vi "XYZ Stage-Command request module.vi"(8 "error in":errorcluster, 9 "Command":T2=enum."Initialize", 11 "XYZ Stage data to queue":T1={"Command"=enum."Initialize", "Channel"="Z", "X"=0.0, "Y"=0.0, "Z"=0.0, "Speed"=0, "Zero"=FALSE, "Use acknowledgement?"=TRUE} {"Speed" format="Speed= %.0f"; "Z" format="Z= %#_g"; "Y" format="Y= %#_g"; "X" format="X= %#_g"}) -> (0 "error out":errorcluster, 1 "Timed out while waiting for acknowledgement":bool, 2 "Dequeue timed out":bool, 3 "XYZ Stage dequeued data":T1={"Command"=enum."Initialize", "Channel"="Z", "X"=0.0, "Y"=0.0, "Z"=0.0, "Speed"=0, "Zero"=FALSE, "Use acknowledgement?"=TRUE} {"Speed" format="Speed= %.0f"; "Z" format="Z= %#_g"; "Y" format="Y= %#_g"; "X" format="X= %#_g"}, 4 "Acknowledgement message":string)   [LabVIEW 2013]
doc: "This is the interface module handling all inter-process signaling between the main software and the XYZ stage driver."
uses:
  Typedefs/XYZ stage data.ctl
  Typedefs/XYZ stage states.ctl
  Typedefs/XYZ channel ring.ctl
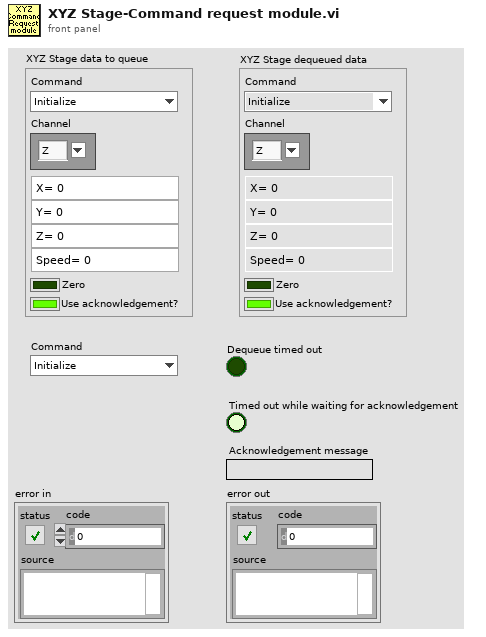
[diagram p1: front panel]
types:
  T1 = typedef "XYZ stage data.ctl" = cluster{"Command":T2, "Channel":T3, "X":sgl, "Y":sgl, "Z":sgl, "Speed":i32, "Zero":bool, "Use acknowledgement?":bool}
  T2 = typedef "XYZ stage states.ctl" = enum16{"Dequeue", "Initialize", "Read Position", "Read Speed Setting", "Move", "Set Max Speed", "Reset Axis", "Stop all movement"}
  T3 = typedef "XYZ channel ring.ctl" = string
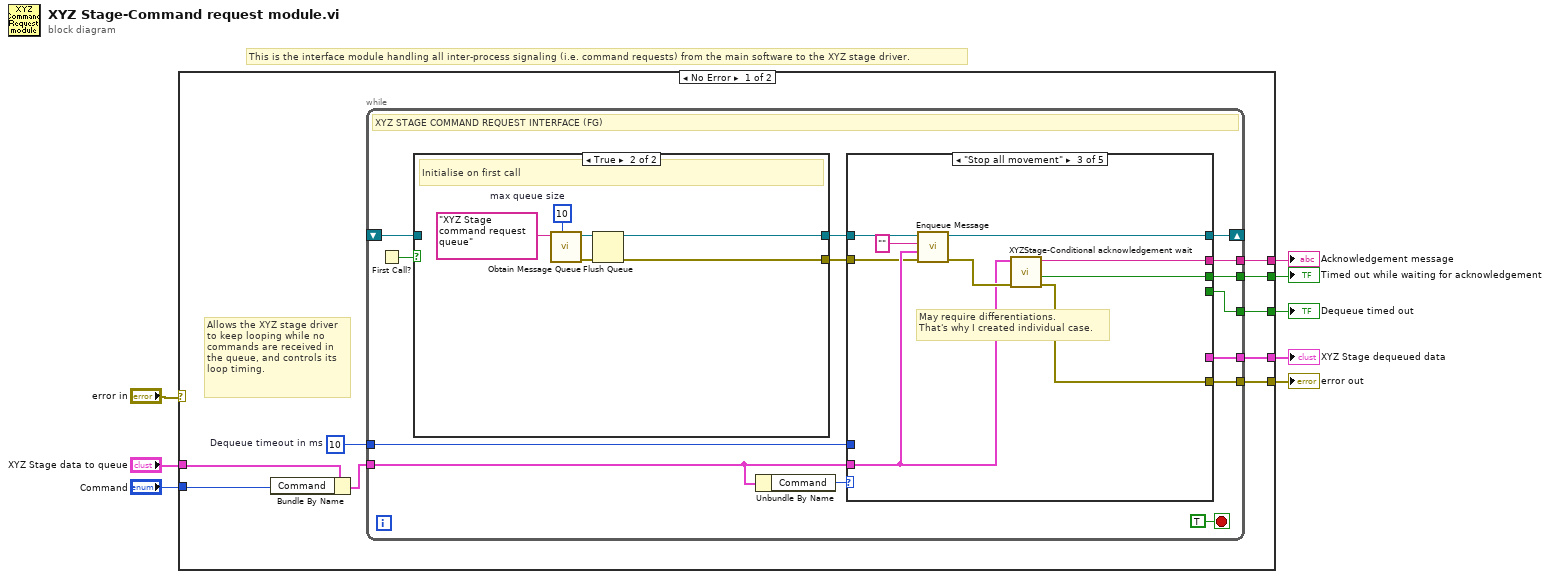
[diagram p0: block diagram]
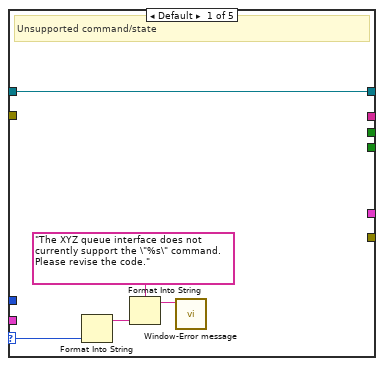
[diagram p2: hidden frame]
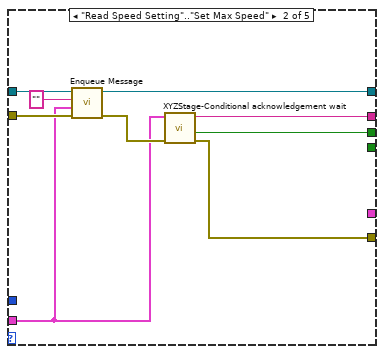
[diagram p3: hidden frame]
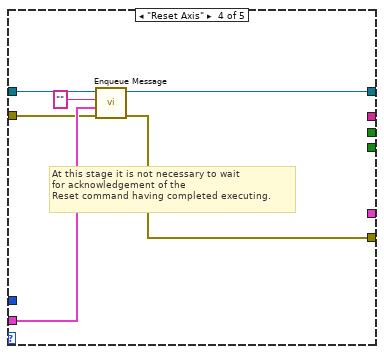
[diagram p4: hidden frame]
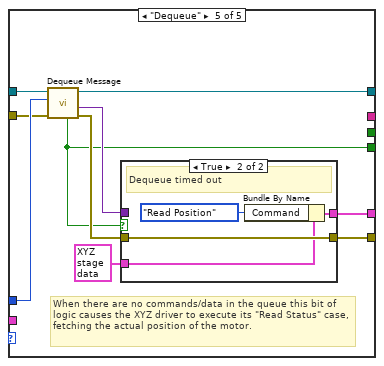
[diagram p5: hidden frame]
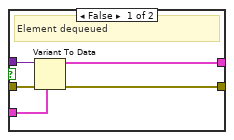
[diagram p6: hidden frame]
diagram:
  # "This is the interface module handling all inter-process signaling (i.e. command requests) from the main software to the XYZ stage driver."
  n1 = case shown="No Error" "error in" {
    selector: "error in" -> [_ w87]
    tunnel: "XYZ Stage data to queue" -> [w16 _]
    tunnel: "Command" -> [w15 _]
    tunnel: [w14 _] -> w6
    tunnel: [w13 _] -> w5
    tunnel: [w12 w87] -> w4
    tunnel: [w11 _] -> w2
    tunnel: [w10 _] -> w1
    frame No Error {
      w9 = 10  # Dequeue timeout in ms
      # "Allows the XYZ stage driver to keep looping while no commands are received in the queue, and controls its loop timing."
      n2 = Bundle By Name(cluster=w16, "Command"=w15) -> (w17:T1)
      n3 = while {
        shift-right: [w25] -> _
        shift-left: _ -> [w29]
        tunnel: w17 -> [w26]
        tunnel: [w24] -> w14
        tunnel: [w23] -> w13
        tunnel: w9 -> [w22]
        tunnel: [w20] -> w12
        tunnel: [w19] -> w11
        tunnel: [w18] -> w10
        stop <- TRUE stop-if-true
        # "XYZ STAGE COMMAND REQUEST INTERFACE (FG)"
        n4 = First Call?() -> (First Call?: T/F=w30:bool)
        n5 = case shown="True" w30 {
          tunnel: [w80 w83] -> w28
          tunnel: w29 -> [w80 _]
          tunnel: [_ w82] -> w21
          frame False {
          }
          frame True {
            w84 = 10  # max queue size
            # "Initialise on first call"
            n6 = call "Obtain Message Queue.vi"("max queue size (-1, unlimited)"=w84, "Queue name"="XYZ Stage command request queue") -> ("error out"=w85:errorcluster, "Message Queue"=w86:refnum<queue>)  [unwired: 8 in]
            n7 = Flush Queue(queue=w86, error in (no error)=w85) -> (queue out=w83:refnum<queue>, error out=w82:errorcluster)  [unwired: 1 out]
          }
        }
        n8 = Unbundle By Name(w26) -> ("Command"=w27:T2)
        n9 = case shown="\"Stop all movement\"" w27 {
          selector: w27 -> [w35 _ _ _ _]
          tunnel: w28 -> [w36 w45 w47 w60 w70]
          tunnel: w26 -> [_ w38 w49 w59 _]
          tunnel: [w36 w44 w54 w58 w68] -> w25
          tunnel: [_ _ _ _ w61] -> w24
          tunnel: [_ _ _ _ w62] -> w23
          tunnel: w22 -> [_ _ _ _ w67]
          tunnel: w21 -> [_ w42 w46 w56 w66]
          tunnel: [_ w40 w51 w55 w64] -> w20
          tunnel: [_ w37 w48 _ _] -> w19
          tunnel: [_ w39 w50 _ _] -> w18
          frame Default {
            # "Unsupported command/state"
            n10 = Format Into String(w35) -> (resulting string=w33:string)  [unwired: 3 in, 1 out]
            n11 = Format Into String(format string="The XYZ queue interface does not currently support the \"%s\" command. Please revise the code.", w33) -> (resulting string=w32:string)  [unwired: 2 in, 1 out]
            n12 = call "Window-Error message.vi"("Message"=w32) -> ()  [unwired: 10 in, 1 out]
          }
          frame "Read Speed Setting".."Set Max Speed" {
            n13 = call "Enqueue Message.vi"("error in (no error)"=w42, "Message Data"=w38, "Message"="", "Queue"=w45) -> ("error out"=w41:errorcluster, "Queue out"=w44:refnum<queue>)  [unwired: 6 in]
            n14 = call "XYZStage-Conditional acknowledgement wait.vi"("error in (no error)"=w41, "XYZ Stage data to queue"=w38) -> ("error out"=w40:errorcluster, "Timed out while waiting for acknowledgement"=w37:bool, "Acknowledgement Message out"=w39:string)  [unwired: 7 in]
          }
          frame "Stop all movement" {
            # "May require differentiations.\nThat's why I created individual case."
            n15 = call "Enqueue Message.vi"("error in (no error)"=w46, "Message Data"=w49, "Message"="", "Queue"=w47) -> ("error out"=w52:errorcluster, "Queue out"=w54:refnum<queue>)  [unwired: 6 in]
            n16 = call "XYZStage-Conditional acknowledgement wait.vi"("error in (no error)"=w52, "XYZ Stage data to queue"=w49) -> ("error out"=w51:errorcluster, "Timed out while waiting for acknowledgement"=w48:bool, "Acknowledgement Message out"=w50:string)  [unwired: 7 in]
          }
          frame "Reset Axis" {
            # "At this stage it is not necessary to wait \nfor acknowledgement of the\nReset command having completed executing."
            n17 = call "Enqueue Message.vi"("error in (no error)"=w56, "Message Data"=w59, "Message"="", "Queue"=w60) -> ("error out"=w55:errorcluster, "Queue out"=w58:refnum<queue>)  [unwired: 6 in]
          }
          frame "Dequeue" {
            # "When there are no commands/data in the queue this bit of logic causes the XYZ driver to execute its \"Read Status\" case, fetching the actual position of the motor."
            n18 = call "Dequeue Message.vi"("Error In"=w66, "timeout in ms (-1)"=w67, "Message Queue"=w70) -> ("Error Out"=w65:errorcluster, "Message Data"=w69:variant, "dup Message Queue"=w68:refnum<queue>, "timed out?"=w61:bool)  [unwired: 4 in, 1 out]
            n19 = case shown="True" w61 {
              tunnel: w69 -> [w75 _]
              tunnel: w65 -> [w74 w77]
              tunnel: [w73 w77] -> w64
              tunnel: [w72 w78] -> w62
              tunnel: T1 {"Command"=enum."Initialize", "Channel"="", "X"=0.0, "Y"=0.0, "Z"=0.0, "Speed"=0, "Zero"=FALSE, "Use acknowledgement?"=FALSE} ("XYZ Stage data to queue") -> [w71 w76]
              frame False {
                # "Element dequeued"
                n20 = Variant To Data(error in=w74, type=w71, Variant=w75) -> (data=w72:T1, error out=w73:errorcluster)
              }
              frame True {
                # "Dequeue timed out"
                n21 = Bundle By Name(cluster=w76, "Command"=XYZ_stage_states."Read Position" ("XYZStageMode")) -> (w78:T1)
              }
            }
          }
        }
      }
    }
    frame Error {
    }
  }
  "Dequeue timed out" <- w6
  "XYZ Stage dequeued data" <- w5
  "error out" <- w4
  "Timed out while waiting for acknowledgement" <- w2
  "Acknowledgement message" <- w1
